vi "LaguerrePolynomialLUTLookup.vi"(1 "x":dbl, 2 "Look-up Table":T1) -> (0 "Function value":dbl)   [LabVIEW 2024]
doc: "This takes the LUT generated by either LaguerreGaussLUTGenerate or LaguerrePolynomialLUTGenerate and looks up the value of the polynomial for EITHER x^2 (LaguerreGauss) OR 2x^2 (LaguerrePolynomial). The factor of two is there to retain interchangeability with the LaguerrePolynomial VI."
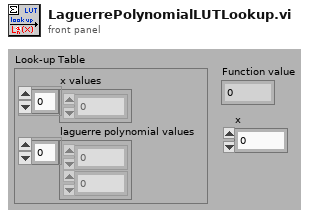
[diagram p1: front panel]
types:
  T1 = cluster{"x values":dbl[], "laguerre polynomial values":dbl[]}
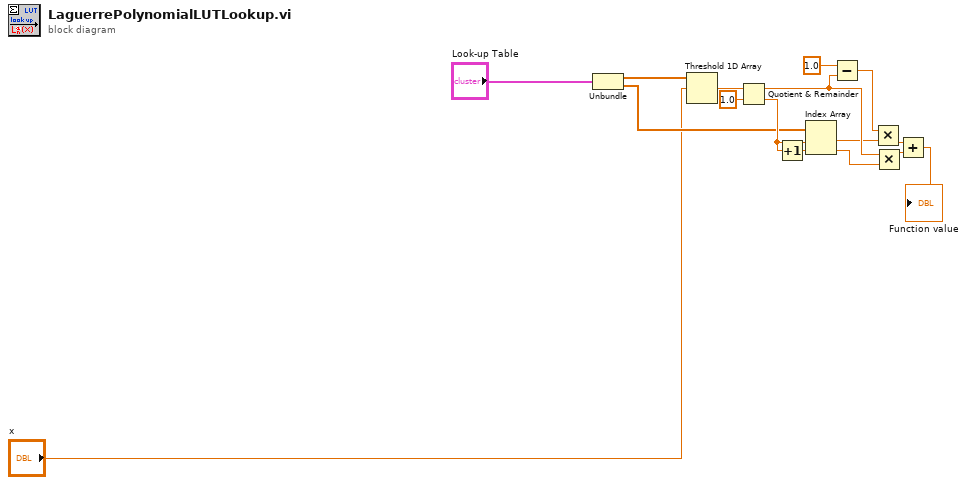
[diagram p0: block diagram]
diagram:
  n1 = Unbundle("Look-up Table") -> ("x values"=w3:dbl[], "laguerre polynomial values"=w6:dbl[])
  n2 = Threshold 1D Array(2:"x", 3:w3) -> (0:w1:dbl)  [unwired: 1 in]
  n3 = Quotient & Remainder(x=w1, y=1.0) -> (x-y*floor(x/y)=w13:dbl, floor(x/y)=w8:dbl)
  n4 = Increment(x=w8) -> (x+1=w7:dbl)
  n5 = Index Array(array=w6, index #1=w8, index #2=w7) -> (element #1=w11:dbl, element #2=w12:dbl)
  n6 = Subtract(x=1.0, y=w13) -> (x-y=w10:dbl)
  n7 = Multiply(x=w10, y=w11) -> (x*y=w14:dbl)
  n8 = Multiply(x=w13, y=w12) -> (x*y=w15:dbl)
  n9 = Add(x=w14, y=w15) -> (x+y=→"Function value":dbl)
